vi "AddControlToControlStateArray.vi"(8 "error in (no error)":errorcluster, 10 "Ctl Refnum":refnum<vi>, 11 "Control State Array":T1[](array[typedef])) -> (0 "error out":errorcluster, 3 "Control State Array (out)":T1[](array[typedef]))   [LabVIEW 2017]
doc: "Adds new control reference to array of control states. States are: Visible (T/F), Enabled (Enabled, Disabled, Disabled and greyed out)"
uses:
  Types/ControlAttributes.ctl
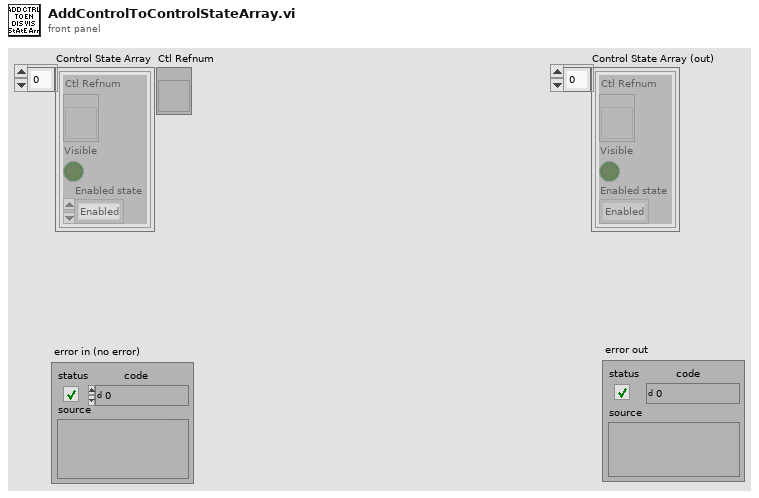
[diagram p1: front panel]
types:
  T1 = typedef "ControlAttributes.ctl" = cluster{"Ctl Refnum":refnum<vi>, "Visible":bool, "Enabled state":enum8{"Enabled", "Disabled", "Disabled and Grayed Out"}}
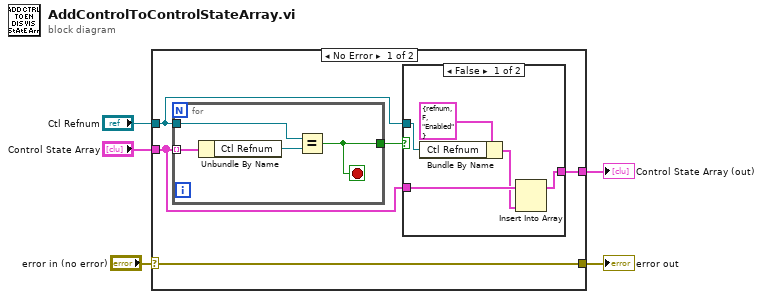
[diagram p0: block diagram]
diagram:
  n1 = case shown="No Error" "error in (no error)" {
    selector: "error in (no error)" -> [w10 w22]
    tunnel: [w10 w22] -> w4
    tunnel: "Control State Array" -> [w8 w21]
    tunnel: "Ctl Refnum" -> [w6 _]
    tunnel: [w9 w21] -> w1
    frame No Error {
      n2 = for {
        tunnel: w8 -> [w19] mode=indexing
        tunnel: w6 -> [w17]
        tunnel: [w18] -> w7
        stop <- w18 stop-if-true
        n3 = Unbundle By Name(w19) -> ("Ctl Refnum"=w20:refnum<vi>)
        n4 = Equal?(x=w17, y=w20) -> (x = y?=w18:bool)
      }
      n5 = case shown="False" w7 {
        tunnel: [w15 w16] -> w9
        tunnel: w8 -> [w14 w16]
        tunnel: w6 -> [w11 _]
        frame False {
          n6 = Bundle By Name(cluster=T1 {"Ctl Refnum"=refnum, "Visible"=FALSE, "Enabled state"=enum."Enabled"} ("Control Attributes"), "Ctl Refnum"=w11) -> (w12:T1)
          n7 = Insert Into Array(array=w14, new element=w12) -> (w15:T1[])  [unwired: 1 in]
        }
        frame True {
        }
      }
    }
    frame Error {
    }
  }
  "error out" <- w4
  "Control State Array (out)" <- w1
